vi "createCamera.vi"(8 "error in (no error)":errorcluster, 9 "machine name":string, 10 "Camera":string, 11 "NetworkCamera in":refnum<class "NetworkCamera.lvclass">) -> (0 "error out":errorcluster, 3 "NetworkCamera out":refnum<class "NetworkCamera.lvclass">)   [LabVIEW 2011, in "Hardware.lvlib" / "HWControllers.lvlib" / "NetworkCamera.lvclass"]
uses:
  NetworkCamera.lvclass
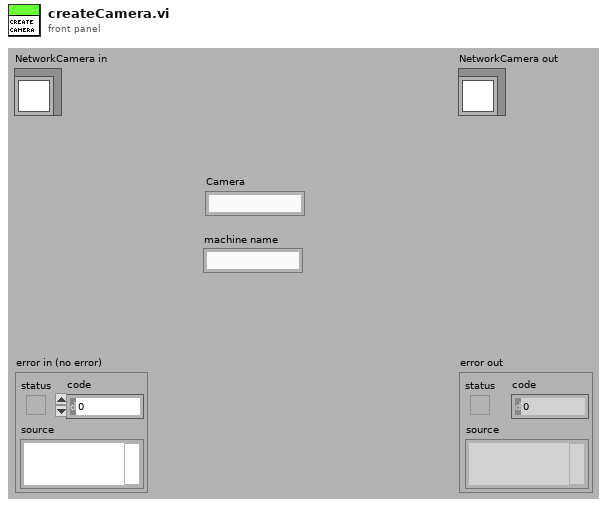
[diagram p1: front panel]
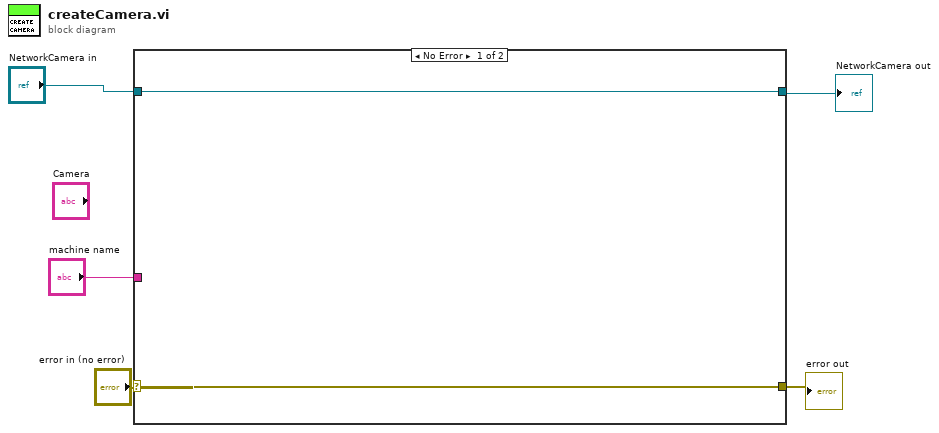
[diagram p0: block diagram]
diagram:
  n1 = case shown="No Error" "error in (no error)" {
    selector: "error in (no error)" -> [w7 w8]
    tunnel: [w6 w9] -> w1
    tunnel: "NetworkCamera in" -> [w6 w9]
    tunnel: [w7 w8] -> w4
    tunnel: "machine name" -> [_ _]
    frame No Error {
    }
    frame Error {
    }
  }
  "error out" <- w4
  "NetworkCamera out" <- w1
